vi "LU Factorization.vi"   [LabVIEW 2012, in "NI_AALPro.lvlib"]
doc: "Performs the LU factorization of <B>A</B> so that <B>PA</B> = <B>LU</B>. Wire data to the <B>A</B> input to determine the polymorphic instance to use or manually select the instance."
uses:
  NI_AALPro.lvlib
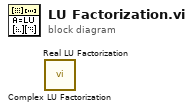
[diagram p0: block diagram]
diagram:
  n1 = call "Complex LU Factorization.vi"() -> ()  [unwired: 1 in, 4 out]
  n2 = call "Real LU Factorization.vi"() -> ()  [unwired: 1 in, 4 out]
